vi "SetBiasAH2550.vi"(8 "error in (no error)":errorcluster, 9 "Bias (Off)":i32(ring) items=["Disabled", "100 megohm", "1 megohm"], 10 "V/A ?":enum16{"DC V"}(ring), 11 "On/Off":bool) -> (0 "error out":errorcluster)   [LabVIEW 2009]
uses:
  Instance           1 15Saved   SetBias .vi
  Instance           2 15Saved   SetBias .vi
  <instrlib>/Andeen-Hagerling 2550/Andeen-Hagerling 2550.lvlib
panel:
  # "On: Bias einschalten\nOff: Bias ausschalten"
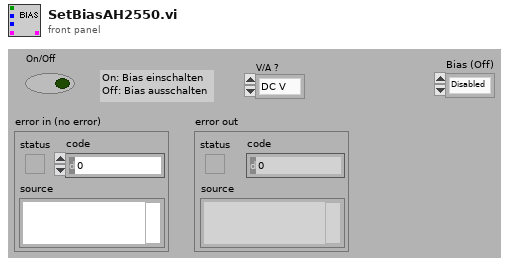
[diagram p1: front panel]
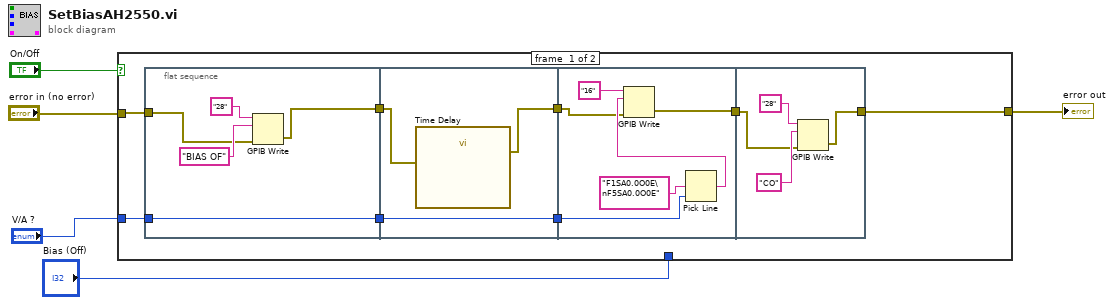
[diagram p0: block diagram]
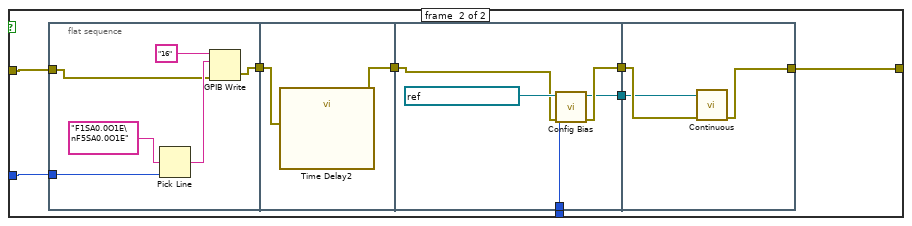
[diagram p2: hidden frame]
diagram:
  n1 = case shown="True" "On/Off" {
    tunnel: "error in (no error)" -> [w12 w39]
    tunnel: "V/A ?" -> [w13 w38]
    tunnel: [w9 w33] -> w2
    tunnel: "Bias (Off)" -> [_ w32]
    frame #0 {
      n2 = flat-sequence {
        tunnel: w13 -> [w15]
        tunnel: w12 -> [w16]
        tunnel: [w14] -> w11
        tunnel: [w15] -> w7
        tunnel: w11 -> [w21]
        tunnel: [w20] -> w10
        tunnel: [w19] -> w8
        tunnel: w7 -> [w19]
        tunnel: w10 -> [w23]
        tunnel: w8 -> [w22]
        tunnel: [w24] -> w6
        tunnel: [w29] -> w9
        tunnel: w6 -> [w30]
        frame #0 {
          n3 = GPIB Write(0:"28", 1:"BIAS OF", 3:w16) -> (6:w14:errorcluster)  [unwired: 2 in, 1 out]
        }
        frame #1 {
          n4 = call "Time Delay"("error in (no error)"=w21) -> ("error out"=w20:errorcluster)  [unwired: 10 in]
        }
        frame #2 {
          n5 = Pick Line(multi-line string="F1SA0.0O0E\nF5SA0.0O0E", line index=w22) -> (output string=w25:string)  [unwired: 1 in]
          n6 = GPIB Write(0:"16", 1:w25, 3:w23) -> (6:w24:errorcluster)  [unwired: 2 in, 1 out]
        }
        frame #3 {
          n7 = GPIB Write(0:"28", 1:"CO", 3:w30) -> (6:w29:errorcluster)  [unwired: 2 in, 1 out]
        }
      }
    }
    frame #1 {
      n8 = flat-sequence {
        tunnel: w39 -> [w40]
        tunnel: w38 -> [w42]
        tunnel: [w41] -> w37
        tunnel: w37 -> [w47]
        tunnel: [w46] -> w36
        tunnel: w36 -> [w51]
        tunnel: [w50] -> w35
        tunnel: [w49] -> w34
        tunnel: w32 -> [w48]
        tunnel: w35 -> [w55]
        tunnel: w34 -> [w54]
        tunnel: [w53] -> w33
        frame #0 {
          n9 = Pick Line(multi-line string="F1SA0.0O1E\nF5SA0.0O1E", line index=w42) -> (output string=w45:string)  [unwired: 1 in]
          n10 = GPIB Write(0:"16", 1:w45, 3:w40) -> (6:w41:errorcluster)  [unwired: 2 in, 1 out]
        }
        frame #1 {
          n11 = call "Time Delay2"("error in (no error)"=w47) -> ("error out"=w46:errorcluster)  [unwired: 10 in]
        }
        frame #2 {
          n12 = call <instrlib>:"Config Bias.vi"("error in"=w51, "Bias (Off)"=w48, "VISA resource name"=refnum<visa-resource-name> "GPIB0::28::INSTR") -> ("error out"=w50:errorcluster, "VISA resource name out"=w49:refnum<visa-resource-name>)  [unwired: 7 in]
        }
        frame #3 {
          n13 = call <instrlib>:"Continuous.vi"("error in"=w55, "VISA resource name"=w54) -> ("error out"=w53:errorcluster)  [unwired: 8 in, 1 out]
        }
      }
    }
  }
  "error out" <- w2
